vi "GetCyclicDataMVP15.vi"(8 "error In":errorcluster, 9 "Map In":map{T1, variant}(c390), 10 "Adress":u16=1 max=999 step=1, 11 "VISA session":refnum<visa-resource-name>) -> (0 "error out":errorcluster, 2 "Map":map{T1, variant}(c390), 3 "VISA session Out":refnum<visa-resource-name>)   [LabVIEW 2019]
uses:
  PfeifferMVP15Cmds.ctl
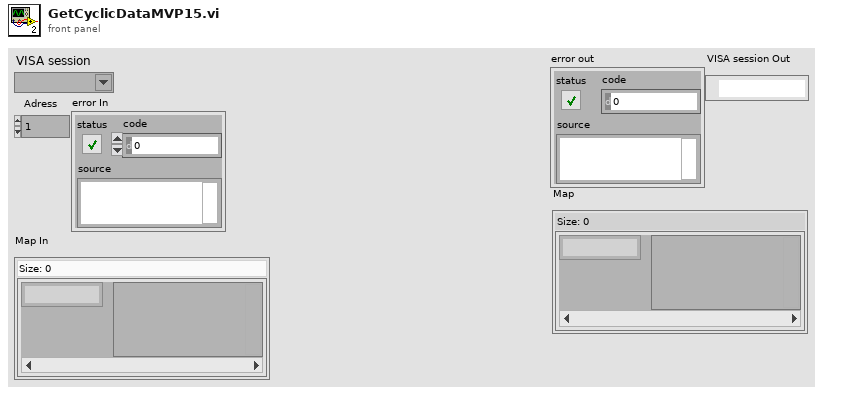
[diagram p1: front panel]
types:
  T1 = typedef "PfeifferMVP15Cmds.ctl" = enum16{"Standby", "Run", "AckError", "ErrorCode", "ActualSpdHz", "DrvCurrent", "OpHrsPump", "FwVersion", "DrvVoltage", "NominalSpdHz", "DrvPower", "ElecName", "HWVersion", "ActualSpdRPM", "NominalSpdRPM", "TempPump"}
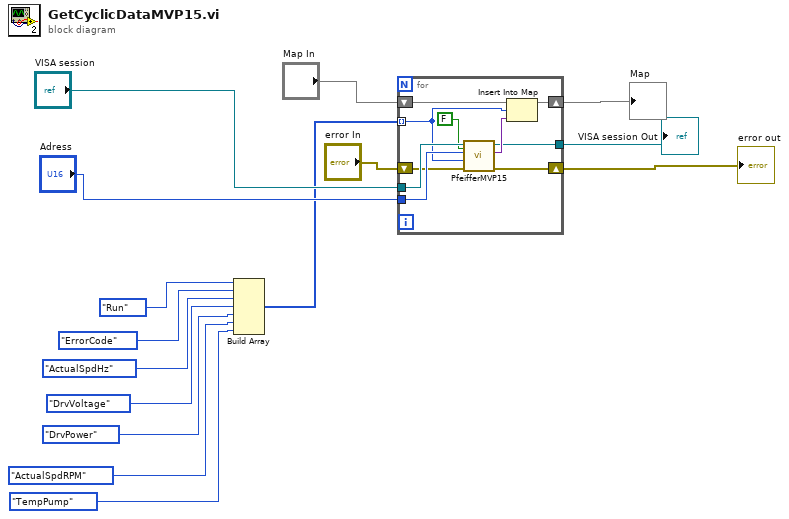
[diagram p0: block diagram]
diagram:
  n1 = Build Array(PfeifferMVP15Cmds."Run" ("Cmd"), PfeifferMVP15Cmds."ErrorCode" ("Cmd"), PfeifferMVP15Cmds."ActualSpdHz" ("Cmd"), PfeifferMVP15Cmds."DrvVoltage" ("Cmd"), PfeifferMVP15Cmds."DrvPower" ("Cmd"), PfeifferMVP15Cmds."ActualSpdRPM" ("Cmd"), PfeifferMVP15Cmds."TempPump" ("Cmd")) -> (w6:T1[])
  n2 = for {
    tunnel: "VISA session" -> [w25]
    tunnel: "Adress" -> [w24]
    tunnel: w6 -> [w22] mode=indexing
    shift-right: [w20] -> w4
    shift-left: "Map In" -> [w19]
    shift-right: [w18] -> w5
    shift-left: "error In" -> [w17]
    tunnel: [w16] -> w1
    n3 = call "PfeifferMVP15.vi"("Write?"=FALSE, "error in"=w17, "Cmd"=w22, "Adress"=w24, "VISA session"=w25) -> ("error out"=w18:errorcluster, "Result"=w21:variant, "VISA session Out"=w16:refnum<visa-resource-name>)  [unwired: 4 in]
    n4 = Insert Into Map(map in=w19, key=w22, value=w21) -> (map out=w20:map{T1, variant})  [unwired: 2 out]
  }
  "error out" <- w5
  "Map" <- w4
  "VISA session Out" <- w1
